vi "Conf Scan.vi"(0 "VISA Resource Name":refnum<visa-resource-name>, 1 "Set/Check (F:Set)":bool, 2 "Check Parameter (0:Ch Delay)":T2(ring), 5 "Time Type (F:Absolute)":bool, 7 "Auto Channel Delay? (F:Off)":bool, 9 "Channel Delay (0 sec)":dbl min=0.0 max=60.0 format="%.2f", 11 "error in (no error)":errorcluster, 12 "Channel List (empty)":string, 13 "Scan Fields":T1) -> (4 "VISA Resource Name Out":refnum<visa-resource-name>, 8 "Configuration?":string, 15 "error out":errorcluster)   [LabVIEW 2012, in "Agilent 34970.lvlib"]
doc: "This VI lets you set or check the scan configuration for selected channels.\n\nThis is an advanced configuration VI. For more information on the different ways to take and configure a measurment, refer to the context help and block diagram of \"HP34970A Advanced Scan Example.vi\"."
uses:
  <instrlib>/Agilent 34970/Agilent 34970.lvlib
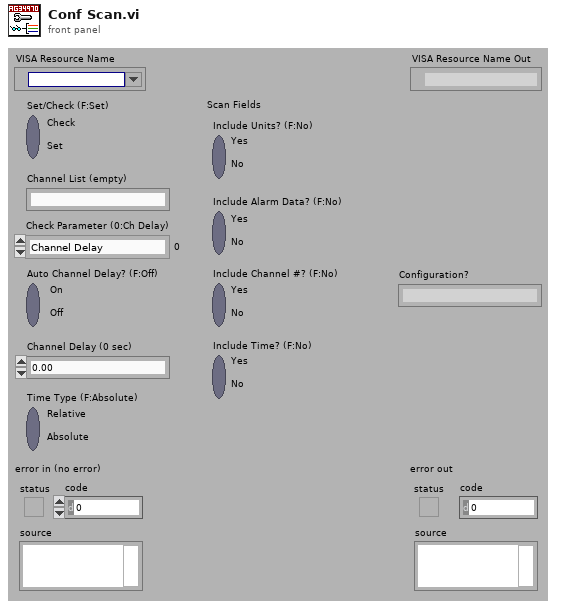
[diagram p1: front panel]
types:
  T1 = cluster{"Include Alarm Data? (F:No)":bool, "Include Channel #? (F:No)":bool, "Include Time? (F:No)":bool, "Include Units? (F:No)":bool}
  T2 = enum16{"Channel Delay", "Auto Delay", "Time Type", "Include Alarm ", "Include Channel", "Include Time", "Include Units", "# Readings", "Time Since Start"}
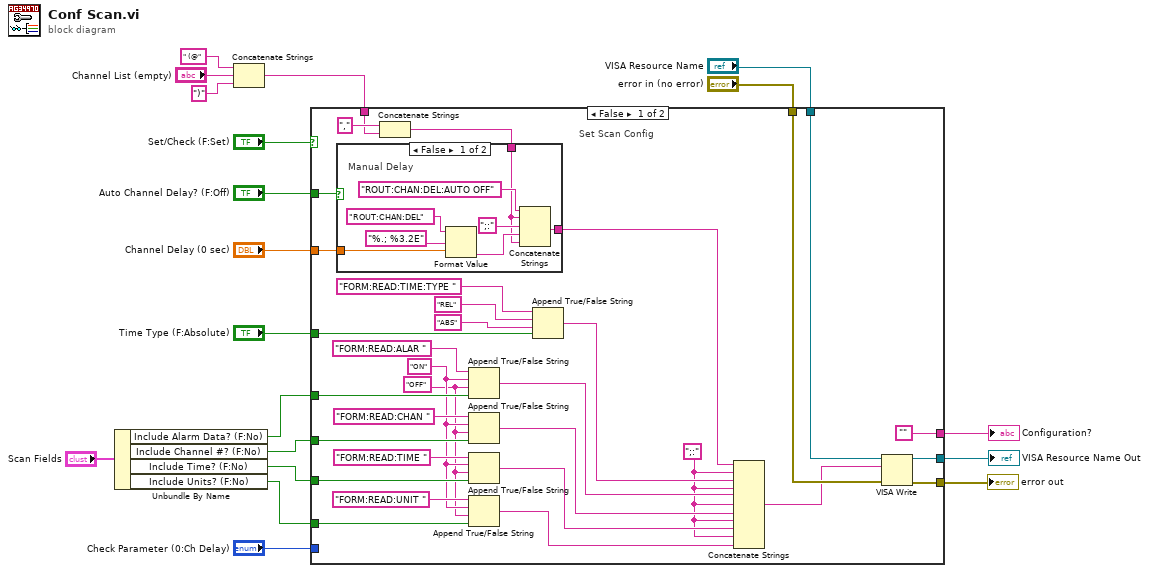
[diagram p0: block diagram]
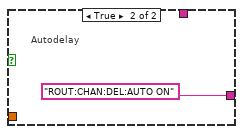
[diagram p2: hidden frame]
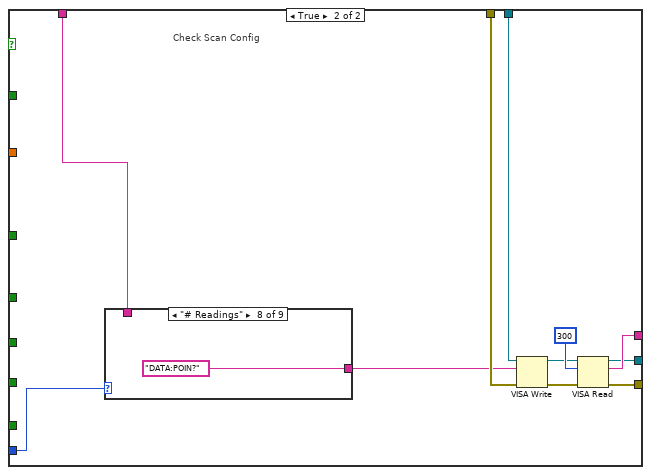
[diagram p3: hidden frame]
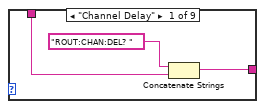
[diagram p4: hidden frame]
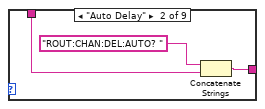
[diagram p5: hidden frame]
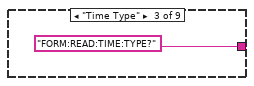
[diagram p6: hidden frame]
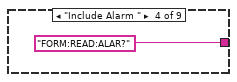
[diagram p7: hidden frame]
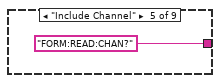
[diagram p8: hidden frame]
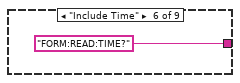
[diagram p9: hidden frame]
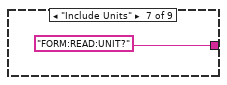
[diagram p10: hidden frame]
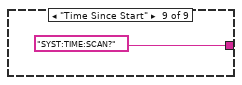
[diagram p11: hidden frame]
diagram:
  n1 = Unbundle By Name("Scan Fields") -> ("Include Alarm Data? (F:No)"=w9:bool, "Include Channel #? (F:No)"=w8:bool, "Include Time? (F:No)"=w7:bool, "Include Units? (F:No)"=w6:bool)
  n2 = Concatenate Strings(" (@", "Channel List (empty)", ")") -> (w16:string)
  n3 = case shown="False" "Set/Check (F:Set)" {
    tunnel: [w47 w71] -> w4
    tunnel: [w48 w68] -> w5
    tunnel: w16 -> [w45 w62]
    tunnel: ["" w69] -> w15
    tunnel: "VISA Resource Name" -> [w50 w67]
    tunnel: "error in (no error)" -> [w49 w66]
    tunnel: "Check Parameter (0:Ch Delay)" -> [_ w63]
    tunnel: "Auto Channel Delay? (F:Off)" -> [w44 _]
    tunnel: "Channel Delay (0 sec)" -> [w43 _]
    tunnel: "Time Type (F:Absolute)" -> [w38 _]
    tunnel: w9 -> [w33 _]
    tunnel: w8 -> [w32 _]
    tunnel: w7 -> [w31 _]
    tunnel: w6 -> [w30 _]
    frame False {
      w22 = ";:"
      w29 = "ON" ("true string")
      w28 = "OFF"
      # "Set Scan Config"
      n4 = Concatenate Strings(",", w45) -> (w42:string)
      n5 = case shown="False" w44 {
        tunnel: w43 -> [w57 _]
        tunnel: w42 -> [w53 _]
        tunnel: [w52 "ROUT:CHAN:DEL:AUTO ON"] -> w27
        frame False {
          # "Manual Delay"
          n6 = Format Value(string ("")="ROUT:CHAN:DEL", format string="%.; %3.2E", value (0)=w57) -> (output string=w54:string)
          n7 = Concatenate Strings("ROUT:CHAN:DEL:AUTO OFF", w53, ";:", w54, w53) -> (w52:string)
        }
        frame True {
          # "Autodelay"
        }
      }
      n8 = Append True/False String(1:w33, 2:w28, 3:w29, 4:"FORM:READ:ALAR ") -> (0:w25:string)
      n9 = Append True/False String(1:w32, 2:w28, 3:w29, 4:"FORM:READ:CHAN ") -> (0:w24:string)
      n10 = Append True/False String(1:w31, 2:w28, 3:w29, 4:"FORM:READ:TIME ") -> (0:w23:string)
      n11 = Append True/False String(1:w30, 2:w28, 3:w29, 4:"FORM:READ:UNIT ") -> (0:w21:string)
      n12 = Append True/False String(1:w38, 2:"ABS", 3:"REL" ("true string"), 4:"FORM:READ:TIME:TYPE ") -> (0:w26:string)
      n13 = Concatenate Strings(w27, w22, w26, w22, w25, w22, w24, w22, w23, w22, w21) -> (w20:string)
      n14 = VISA Write(VISA resource name=w50, write buffer=w20, error in (no error)=w49) -> (VISA resource name out=w48:refnum<visa-resource-name>, error out=w47:errorcluster)  [unwired: 1 out]
    }
    frame True {
      # "Check Scan Config"
      n15 = case shown="\"# Readings\"" w63 {
        tunnel: w62 -> [w74 w75 _ _ _ _ _ _ _]
        tunnel: [w72 w76 "FORM:READ:TIME:TYPE?" "FORM:READ:ALAR?" "FORM:READ:CHAN?" "FORM:READ:TIME?" "FORM:READ:UNIT?" "DATA:POIN?" "SYST:TIME:SCAN?"] -> w61
        frame "Channel Delay" {
          n16 = Concatenate Strings("ROUT:CHAN:DEL? ", w74) -> (w72:string)
        }
        frame "Auto Delay" {
          n17 = Concatenate Strings("ROUT:CHAN:DEL:AUTO? ", w75) -> (w76:string)
        }
        frame "Time Type" {
        }
        frame "Include Alarm " {
        }
        frame "Include Channel" {
        }
        frame "Include Time" {
        }
        frame "Include Units" {
        }
        frame "# Readings" {
        }
        frame "Time Since Start" {
        }
      }
      n18 = VISA Write(VISA resource name=w67, write buffer=w61, error in (no error)=w66) -> (VISA resource name out=w65:refnum<visa-resource-name>, error out=w64:errorcluster)  [unwired: 1 out]
      n19 = VISA Read(VISA resource name=w65, byte count=u32 300 ("byte count (0)"), error in (no error)=w64) -> (VISA resource name out=w68:refnum<visa-resource-name>, read buffer=w69:string, error out=w71:errorcluster)  [unwired: 1 out]
    }
  }
  "Configuration?" <- w15
  "VISA Resource Name Out" <- w5
  "error out" <- w4
